vi "Select HDF5 Dlg Resize.vi"(8 "error in (no error)":errorcluster, 9 "NewBnds":T1, 10 "Display Path?":bool, 11 "Select HDF5 Dlg Items":T2) -> (0 "error out":errorcluster)   [LabVIEW 2017]
uses:
  <vilib>/Utility/miscctls.llb/LVRectTypeDef.ctl
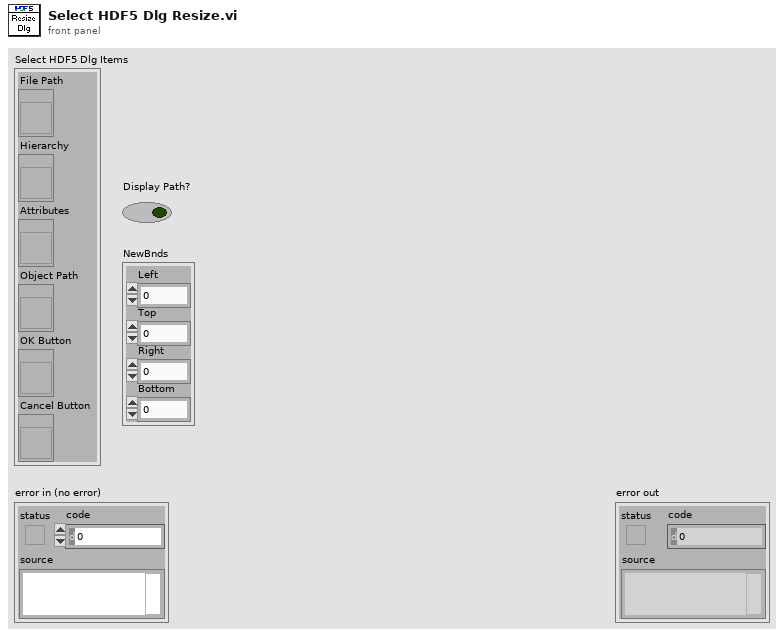
[diagram p1: front panel]
types:
  T1 = typedef "LVRectTypeDef.ctl" = cluster{"Left":i16, "Top":i16, "Right":i16, "Bottom":i16}
  T2 = cluster{"File Path":refnum<vi>, "Hierarchy":refnum<vi>, "Attributes":refnum<vi>, "Object Path":refnum<vi>, "OK Button":refnum<vi>, "Cancel Button":refnum<vi>}
  T3 = typedef "LVBoundsTypeDef.ctl" = cluster{"Width":u32, "Height":u32}
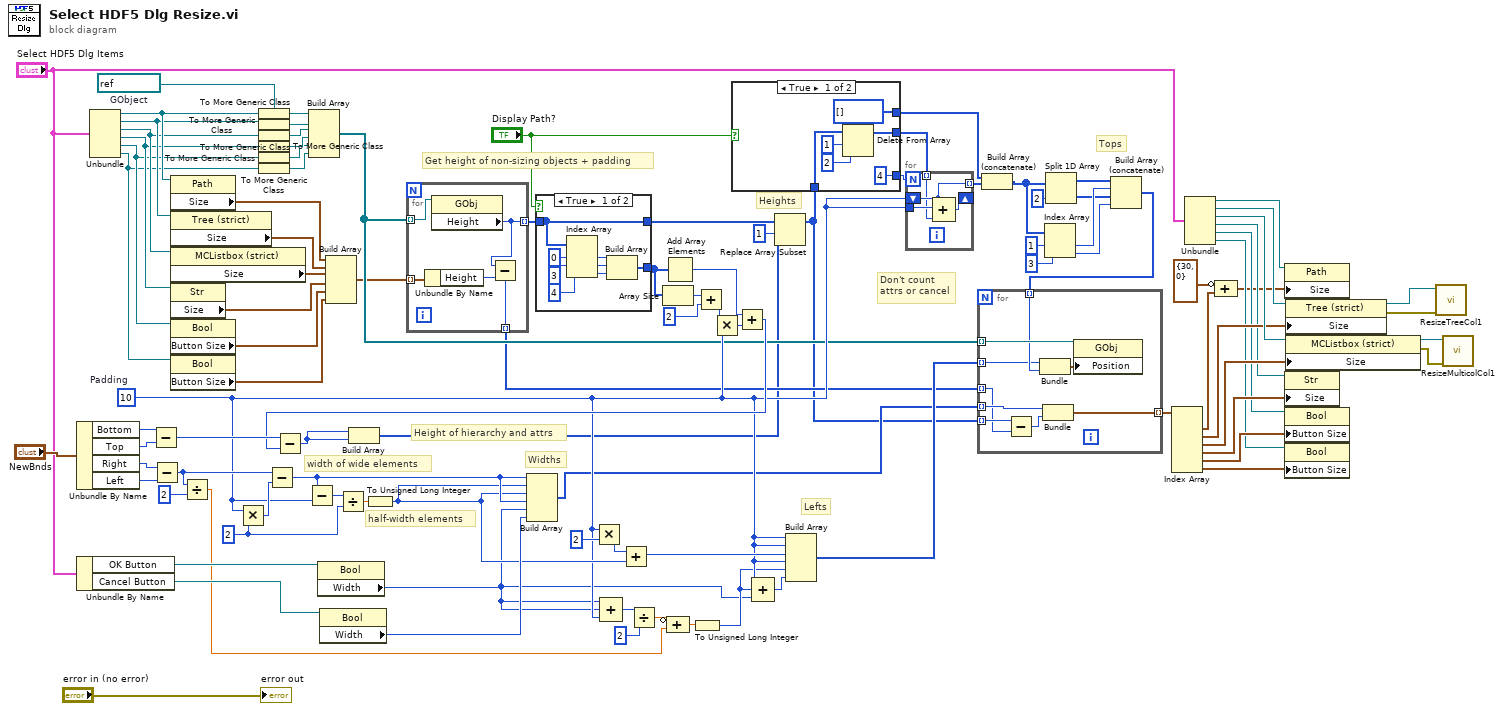
[diagram p0: block diagram]
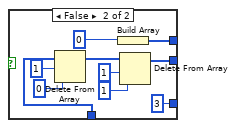
[diagram p2: hidden frame]
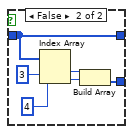
[diagram p3: hidden frame]
diagram:
  w92 = u32 2 ("y")
  w101 = refnum<vi> refnum  # GObject
  w64 = u32 10  # Padding
  # "Don't count\nattrs or cancel"
  # "Lefts"
  # "Tops"
  # "Heights"
  # "Widths"
  # "half-width elements"
  # "width of wide elements"
  # "Height of hierarchy and attrs"
  # "Get height of non-sizing objects + padding"
  n1 = Unbundle By Name("NewBnds") -> ("Bottom"=w99:i16, "Top"=w98:i16, "Right"=w97:i16, "Left"=w96:i16)
  n2 = Unbundle By Name("Select HDF5 Dlg Items") -> ("OK Button"=w89:refnum<vi>, "Cancel Button"=w88:refnum<vi>)
  n3 = Unbundle("Select HDF5 Dlg Items") -> ("File Path"=w36:refnum<vi>, "Hierarchy"=w35:refnum<vi>, "Attributes"=w34:refnum<vi>, "Object Path"=w33:refnum<vi>, "OK Button"=w32:refnum<vi>, "Cancel Button"=w31:refnum<vi>)
  n4 = Subtract(x=w99, y=w98) -> (x-y=w95:i16)
  n5 = Subtract(x=w97, y=w96) -> (x-y=w69:i16)
  n6 = property class="Path"(reference=w36) -> ("Size"=w28:T3)  [unwired: 1 in, 2 out]
  n7 = property class="Tree (strict)"(reference=w35) -> ("Size"=w29:T3)  [unwired: 1 in, 2 out]
  n8 = property class="MCListbox (strict)"(reference=w34) -> ("Size"=w30:T3)  [unwired: 1 in, 2 out]
  n9 = property class="Str"(reference=w33) -> ("Size"=w27:T3)  [unwired: 1 in, 2 out]
  n10 = property class="Bool"(reference=w32) -> ("Button Size"=w26:T3)  [unwired: 1 in, 2 out]
  n11 = property class="Bool"(reference=w31) -> ("Button Size"=w25:T3)  [unwired: 1 in, 2 out]
  n12 = Divide(x=w69, y=i16 2) -> (x/y=w66:dbl)
  n13 = Multiply(x=w64, y=w92) -> (x*y=w94:u32)
  n14 = To More Generic Class(target class=w101, reference=w36) -> (generic class reference=w77:refnum<vi>)
  n15 = To More Generic Class(target class=w101, reference=w35) -> (generic class reference=w76:refnum<vi>)
  n16 = To More Generic Class(target class=w101, reference=w34) -> (generic class reference=w75:refnum<vi>)
  n17 = To More Generic Class(target class=w101, reference=w33) -> (generic class reference=w74:refnum<vi>)
  n18 = To More Generic Class(target class=w101, reference=w32) -> (generic class reference=w73:refnum<vi>)
  n19 = To More Generic Class(target class=w101, reference=w31) -> (generic class reference=w72:refnum<vi>)
  n20 = Subtract(x=w69, y=w94) -> (x-y=w90:u32)
  n21 = Subtract(x=w90, y=w64) -> (x-y=w93:u32)
  n22 = Build Array(w77, w76, w75, w74, w73, w72) -> (w59:refnum<vi>[])
  n23 = property class="Bool"(reference=w89) -> ("Width"=w62:u32)  [unwired: 1 in, 2 out]
  n24 = property class="Bool"(reference=w88) -> ("Width"=w87:u32)  [unwired: 1 in, 2 out]
  n25 = Build Array(w28, w29, w30, w27, w26, w25) -> (w24:T3[])
  n26 = Divide(x=w93, y=w92) -> (x/y=w91:dbl)
  n27 = To Unsigned Long Integer(number=w91) -> (unsigned 32bit integer=w79:u32)
  n28 = for {
    tunnel: w59 -> [w106] mode=indexing
    tunnel: [w103] -> w86 mode=indexing
    tunnel: w24 -> [w105] mode=indexing
    tunnel: [w102] -> w23 mode=indexing
    n29 = Unbundle By Name(w105) -> ("Height"=w104:u32)
    n30 = property class="GObj"(reference=w106) -> ("Height"=w103:u32)  [unwired: 1 in, 2 out]
    n31 = Subtract(x=w103, y=w104) -> (x-y=w102:u32)
  }
  n32 = Build Array(w90, w79, w79, w90, w62, w87) -> (w58:u32[])
  n33 = case shown="True" "Display Path?" {
    tunnel: w86 -> [w107 w115]
    tunnel: [w108 w118] -> w85
    tunnel: [w107 w115] -> w83
    frame True {
      n34 = Index Array(array=w107, index #1=0 ("index"), index #2=3 ("index"), index #3=4 ("index")) -> (element #1=w111:u32, element #2=w110:u32, element #3=w109:u32)
      n35 = Build Array(w111, w110, w109) -> (w108:u32[])
    }
    frame False {
      n36 = Index Array(array=w115, index #1=3 ("index"), index #2=4 ("index")) -> (element #1=w120:u32, element #2=w119:u32)
      n37 = Build Array(w120, w119) -> (w118:u32[])
    }
  }
  n38 = Multiply(x=w64, y=u32 2) -> (x*y=w80:u32)
  n39 = Compound Arithmetic op=ADD(w62, w62, w64) -> (w71:u32)
  n40 = Add(x=w80, y=w79) -> (x+y=w78:u32)
  n41 = Divide(x=w71, y=u32 2) -> (x/y=w67:dbl)
  n42 = Array Size(array=w85) -> (size(s)=w10:i32)
  n43 = Add Array Elements(numeric array=w85) -> (sum=w12:u32)
  n44 = Compound Arithmetic op=ADD(invert w67, w66) -> (w65:dbl)
  n45 = To Unsigned Long Integer(number=w65) -> (unsigned 32bit integer=w63:u32)
  n46 = Add(x=w10, y=2) -> (x+y=w8:i32)
  n47 = Multiply(x=w8, y=w64) -> (x*y=w11:u32)
  n48 = Add(x=w12, y=w11) -> (x+y=w84:u32)
  n49 = Subtract(x=w95, y=w84) -> (x-y=w22:u32)
  n50 = Build Array(w22, w22) -> (w21:u32[])
  n51 = Compound Arithmetic op=ADD(w64, w63, w62) -> (w61:u32)
  n52 = Replace Array Subset(array=w83, new element=w21, index=1) -> (w20:u32[])
  n53 = case shown="True" "Display Path?" {
    tunnel: w20 -> [w124 w132]
    tunnel: [w123 w134] -> w18
    tunnel: [4 3] -> w17
    tunnel: [u32[] [] w127] -> w14
    frame True {
      n54 = Delete From Array(array=w124, length=1, index=2) -> (array with subset deleted=w123:u32[])  [unwired: 1 out]
    }
    frame False {
      n55 = Delete From Array(array=w132, length=1, index=0) -> (array with subset deleted=w131:u32[])  [unwired: 1 out]
      n56 = Build Array(u32 0) -> (w127:u32[])
      n57 = Delete From Array(array=w131, length=1, index=1) -> (array with subset deleted=w134:u32[])  [unwired: 1 out]
    }
  }
  n58 = Build Array(w64, w64, w78, w64, w63, w61) -> (w60:u32[])
  n59 = for {
    N: w17 -> [_]
    shift-right: [w138] -> _
    shift-left: w64 -> [w140]
    tunnel: [w140] -> w15 mode=indexing
    tunnel: w64 -> [w139]
    tunnel: w18 -> [w137] mode=indexing
    n60 = Compound Arithmetic op=ADD(w140, w139, w137) -> (w138:u32)
  }
  n61 = Build Array (concatenate)(w14, w15) -> (w13:u32[])
  n62 = Index Array(array=w13, index #1=1 ("index"), index #2=3 ("index")) -> (element #1=w40:u32, element #2=w38:u32)
  n63 = Split 1D Array(array=w13, index=2) -> (first subarray=w41:u32[], second subarray=w39:u32[])
  n64 = Build Array (concatenate)(w41, w40, w39, w38) -> (w37:u32[])
  n65 = for {
    tunnel: w37 -> [w148] mode=indexing
    tunnel: w60 -> [w147] mode=indexing
    tunnel: w59 -> [w149] mode=indexing
    tunnel: w58 -> [w145] mode=indexing
    tunnel: w20 -> [w143] mode=indexing
    tunnel: [w144] -> w57 mode=indexing
    tunnel: w23 -> [w142] mode=indexing
    n66 = Subtract(x=w143, y=w142) -> (x-y=w141:u32)
    n67 = Bundle("Padding"=w147, "Padding"=w148) -> (w146:cluster{"Padding":u32, "Padding":u32})  [unwired: 1 in]
    n68 = Bundle("Width"=w145, w141) -> (w144:cluster{"Width":u32, u32})  [unwired: 1 in]
    n69 = property class="GObj"(reference=w149, "Position"=w146) -> ()  [unwired: 1 in, 2 out]
  }
  n70 = Index Array(array=w57) -> (element #1=w7:cluster{"Width":u32, u32}, element #2=w49:cluster{"Width":u32, u32}, element #3=w53:cluster{"Width":u32, u32}, element #4=w54:cluster{"Width":u32, u32}, element #5=w55:cluster{"Width":u32, u32}, element #6=w56:cluster{"Width":u32, u32})  [unwired: 6 in]
  n71 = Unbundle("Select HDF5 Dlg Items") -> ("File Path"=w52:refnum<vi>, "Hierarchy"=w51:refnum<vi>, "Attributes"=w50:refnum<vi>, "Object Path"=w48:refnum<vi>, "OK Button"=w47:refnum<vi>, "Cancel Button"=w46:refnum<vi>)
  n72 = Compound Arithmetic op=ADD(invert cluster{"Width":u32, u32} {"Width"=30, 0} ("element"), w7) -> (w5:cluster{"Width":u32, u32})
  n73 = property class="Path"(reference=w52, "Size"=w5) -> ()  [unwired: 1 in, 2 out]
  n74 = property class="Str"(reference=w48, "Size"=w54) -> ()  [unwired: 1 in, 2 out]
  n75 = property class="Bool"(reference=w47, "Button Size"=w55) -> ()  [unwired: 1 in, 2 out]
  n76 = property class="Bool"(reference=w46, "Button Size"=w56) -> ()  [unwired: 1 in, 2 out]
  n77 = property class="Tree (strict)"(reference=w51, "Size"=w49) -> (reference out=w4:refnum<vi>, error out=w3:errorcluster)  [unwired: 1 in]
  n78 = property class="MCListbox (strict)"(reference=w50, "Size"=w53) -> (reference out=w2:refnum<vi>, error out=w1:errorcluster)  [unwired: 1 in]
  n79 = call <vilib>:"ResizeTreeCol1.vi"("error in (no error)"=w3, "TreeControl in"=w4) -> ()  [unwired: 8 in, 2 out]
  n80 = call <vilib>:"ResizeMulticolCol1.vi"("error in (no error)"=w1, "MulticolumnListbox in"=w2) -> ()  [unwired: 8 in, 2 out]
  "error out" <- "error in (no error)"
